vi "CANOpen_Main_Scale RPDO Data.vi"(8 "error in (no error)":errorcluster, 10 "Data":dbl[](array[numeric]), 11 "PDO Settings":T1={"Parameters"=[], "PDO Channel"=1, "Start Index"=0, "Length"=0} {"PDO Channel" items=["PDO 1", "PDO 2", "PDO 3", "PDO 4"]; "Parameters"."Bit Offset" max=8 step=1; "Parameters"."Byte Offset" max=8 step=1}) -> (0 "error out":errorcluster, 3 "CANopen data out":u8[](array[numeric]))   [LabVIEW 2013]
uses:
  Shared Code/CANOpen_PDO Settings.ctl
  Shared Code/CANOpen_PDO Parameter Settings.ctl
  Shared Code/CANOpen_PDO Data Type.ctl
  System Explorer/SubVIs/CANopen Byte Order.ctl
  <vilib>/CANopenLib/CANOPEN.llb/CANopen Convert To Data [U8].vi
  <vilib>/CANopenLib/CANOPEN.llb/CANopen Convert To Data [I8].vi
  <vilib>/CANopenLib/CANOPEN.llb/CANopen Convert To Data [I16].vi
  <vilib>/CANopenLib/CANOPEN.llb/CANopen Convert To Data [I32].vi
  <vilib>/CANopenLib/CANOPEN.llb/CANopen Convert To Data [SGL].vi
  <vilib>/CANopenLib/CANOPEN.llb/CANopen Convert To Data [DBL].vi
  <vilib>/CANopenLib/CANOPEN.llb/CANopen Convert To Data [U16].vi
  <vilib>/CANopenLib/CANOPEN.llb/CANopen Convert To Data [U32].vi
  CANOpen Addon Custom Device.lvlib
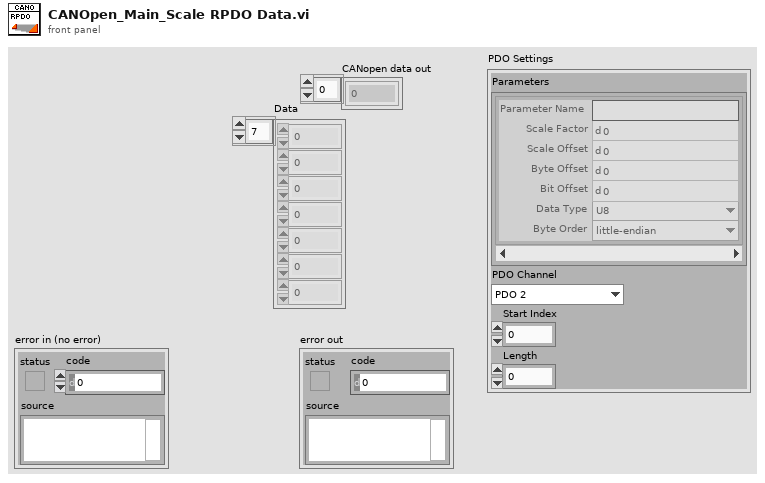
[diagram p1: front panel]
types:
  T1 = typedef "CANOpen Addon Custom Device.lvlib/CANOpen_PDO Settings.ctl" = cluster{"Parameters":T2[], "PDO Channel":u8, "Start Index":u32, "Length":u32}
  T2 = typedef "CANOpen Addon Custom Device.lvlib/CANOpen_PDO Parameter Settings.ctl" = cluster{"Parameter Name":string, "Scale Factor":dbl, "Scale Offset":dbl, "Byte Offset":u8, "Bit Offset":u8, "Data Type":T3, "Byte Order":T4}
  T3 = typedef "CANOpen Addon Custom Device.lvlib/CANOpen_PDO Data Type.ctl" = enum16{"U8", "U16", "U32", "I8", "I16", "I32", "Single", "Double", "Boolean"}
  T4 = typedef "CANOpen Addon Custom Device.lvlib/CANopen Byte Order.ctl" = enum16{"big-endian network order", "little-endian"}
  T5 = enum16{"big-endian, network order", "native, host order", "little-endian"}
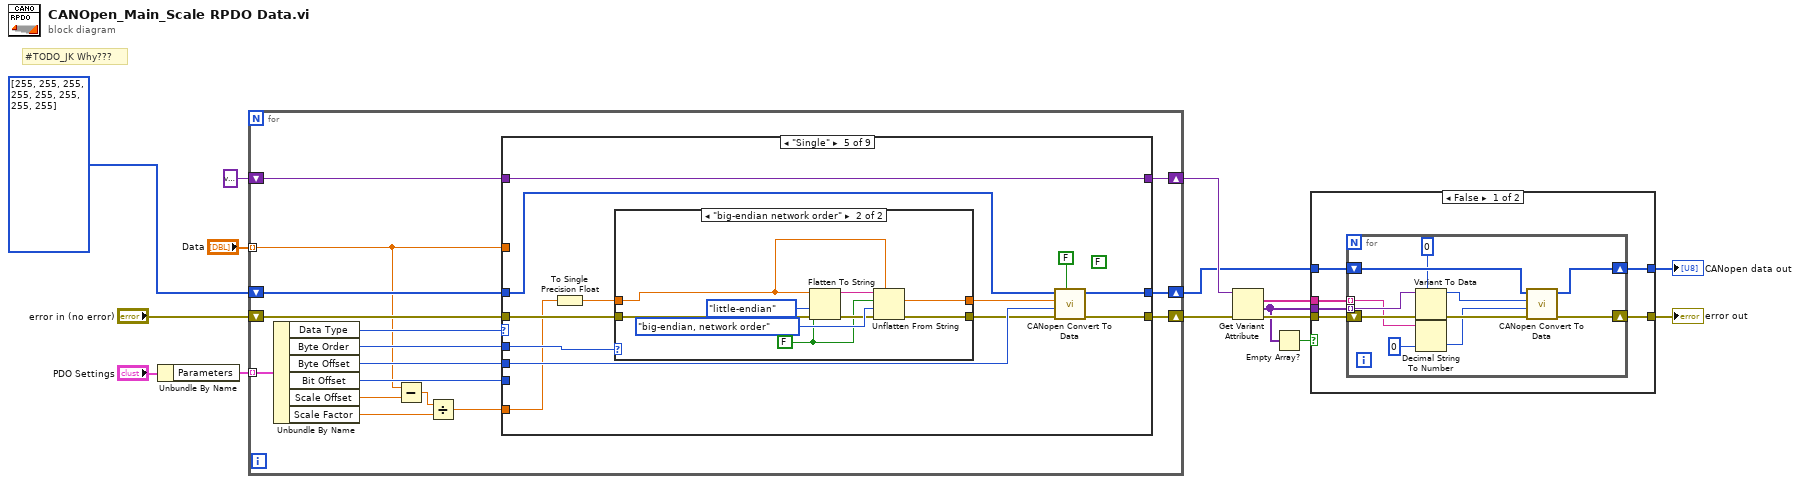
[diagram p0: block diagram]
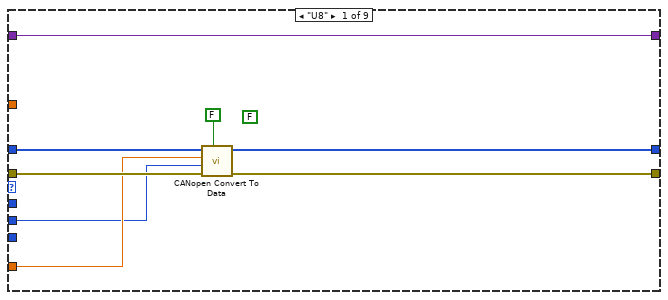
[diagram p3: hidden frame]
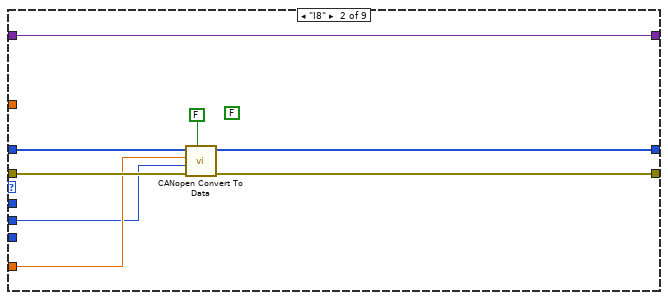
[diagram p4: hidden frame]
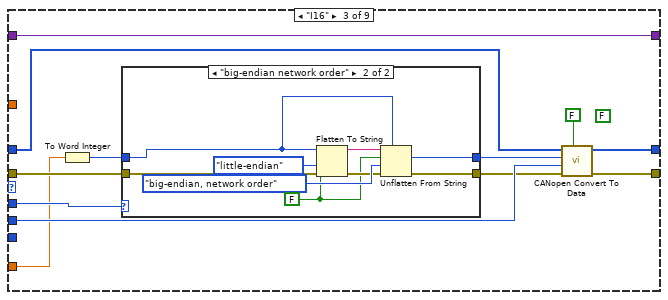
[diagram p5: hidden frame]
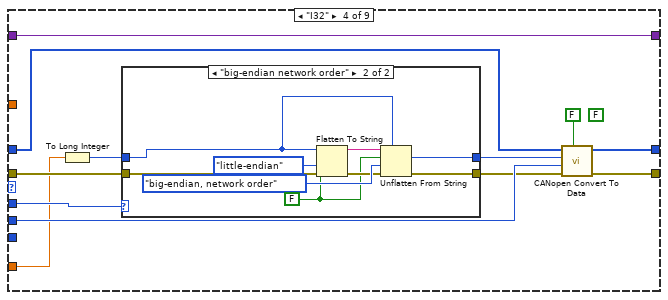
[diagram p7: hidden frame]
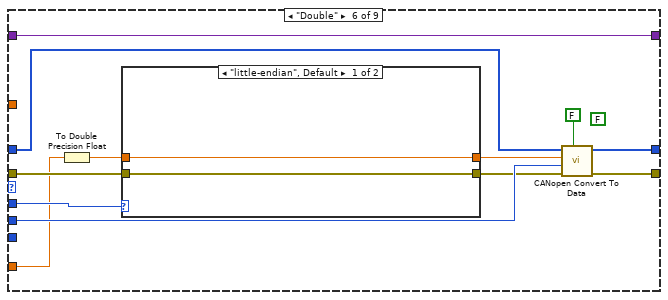
[diagram p10: hidden frame]
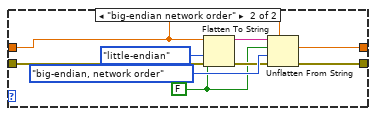
[diagram p11: hidden frame]
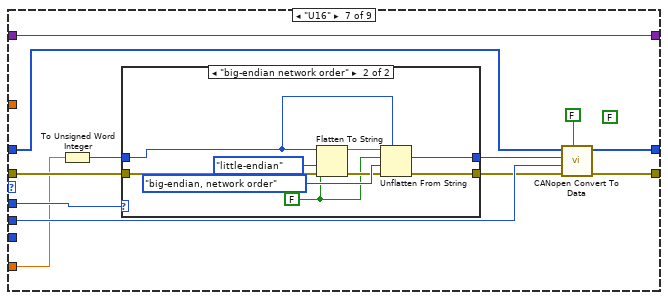
[diagram p12: hidden frame]
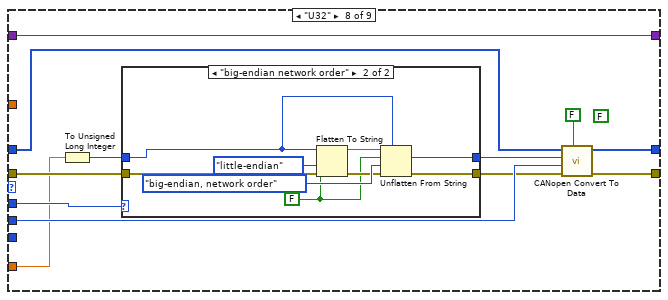
[diagram p14: hidden frame]
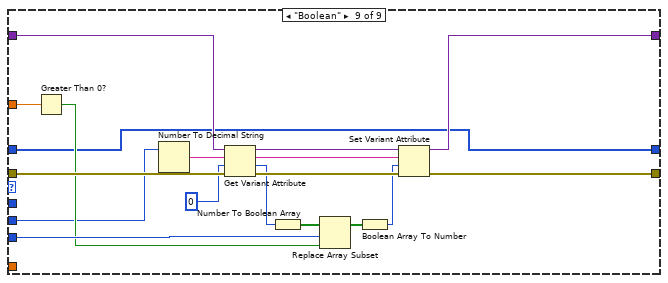
[diagram p16: hidden frame]
diagram:
  # "#TODO_JK Why???"
  n1 = Unbundle By Name("PDO Settings") -> ("Parameters"=w13:T2[])
  n2 = for {
    tunnel: w13 -> [w29] mode=indexing
    shift-right: [w23] -> w5
    shift-left: u8[] [255, 255, 255, 255, 255, 255, 255, 255] ("CANopen data out") -> [w22]
    shift-right: [w31] -> w10
    shift-left: "error in (no error)" -> [w30]
    shift-right: [w18] -> w9
    shift-left: variant ("variant") -> [w19]
    tunnel: "Data" -> [w16] mode=indexing
    n3 = Unbundle By Name(w29) -> ("Data Type"=w24:T3, "Byte Order"=w17:T4, "Byte Offset"=w25:u8, "Bit Offset"=w20:u8, "Scale Offset"=w28:dbl, "Scale Factor"=w21:dbl)
    n4 = Subtract(x=w16, y=w28) -> (x-y=w27:dbl)
    n5 = Divide(x=w27, y=w21) -> (x/y=w26:dbl)
    n6 = case shown="\"Single\"" w24 {
      tunnel: [w39 w47 w59 w82 w105 w128 w151 w174 w199] -> w31
      tunnel: [w37 w45 w57 w80 w103 w126 w149 w172 w189] -> w23
      tunnel: w30 -> [w36 w44 w54 w77 w100 w123 w146 w169 w201]
      tunnel: w26 -> [w35 w43 w49 w72 w95 w118 w141 w164 _]
      tunnel: w25 -> [w34 w42 w56 w79 w102 w125 w148 w171 w188]
      tunnel: w22 -> [w33 w41 w51 w74 w97 w120 w143 w166 w189]
      tunnel: w20 -> [_ _ _ _ _ _ _ _ w194]
      tunnel: w19 -> [w32 w40 w55 w78 w101 w124 w147 w170 w202]
      tunnel: [w32 w40 w55 w78 w101 w124 w147 w170 w190] -> w18
      tunnel: w17 -> [_ _ w52 w75 w98 w121 w144 w167 _]
      tunnel: w16 -> [_ _ _ _ _ _ _ _ w186]
      frame "U8" {
        (unwired) FALSE ("trim")
        n7 = call-poly <vilib>:"CANopen Convert To Data.vi"("trim"=FALSE, "error in (no error)"=w36, "offset (0)"=w34, "unsigned 8-bit integer"=w35, "CANopen data in"=w33) -> ("error out"=w39:errorcluster, "CANopen data out"=w37:u8[])  [unwired: 5 in]
      }
      frame "I8" {
        (unwired) FALSE ("trim")
        n8 = call-poly <vilib>:"CANopen Convert To Data.vi"("trim"=FALSE, "error in (no error)"=w44, "offset (0)"=w42, "signed 8-bit integer"=w43, "CANopen data in"=w41) -> ("error out"=w47:errorcluster, "CANopen data out"=w45:u8[])  [unwired: 5 in]
      }
      frame "I16" {
        (unwired) FALSE ("trim")
        n9 = To Word Integer(number=w49) -> (16bit integer=w50:i16)
        n10 = case shown="\"big-endian network order\"" w52 {
          tunnel: w50 -> [w60 w66]
          tunnel: [w60 w65] -> w48
          tunnel: w54 -> [w61 w64]
          tunnel: [w61 w63] -> w53
          frame "little-endian", Default {
          }
          frame "big-endian network order" {
            w62 = FALSE ("prepend array or string size? (T)")
            n11 = Flatten To String(anything=w66, prepend array or string size? (T)=w62, byte order (0:big-endian, network order)=T5."little-endian", error in (no error)=w64) -> (data string=w69:string, error out=w67:errorcluster)  [unwired: 1 out]
            n12 = Unflatten From String(type=w66, binary string=w69, data includes array or string size? (T)=w62, byte order (0:big-endian, network order)=T5."big-endian, network order", error in (no error)=w67) -> (value=w65:i16, error out=w63:errorcluster)  [unwired: 1 out]
          }
        }
        n13 = call-poly <vilib>:"CANopen Convert To Data.vi"("trim"=FALSE, "error in (no error)"=w53, "offset (0)"=w56, "signed 16-bit integer"=w48, "CANopen data in"=w51) -> ("error out"=w59:errorcluster, "CANopen data out"=w57:u8[])  [unwired: 5 in]
      }
      frame "I32" {
        (unwired) FALSE ("trim")
        n14 = To Long Integer(number=w72) -> (32bit integer=w73:i32)
        n15 = case shown="\"big-endian network order\"" w75 {
          tunnel: w73 -> [w83 w89]
          tunnel: [w83 w88] -> w71
          tunnel: w77 -> [w84 w87]
          tunnel: [w84 w86] -> w76
          frame "little-endian", Default {
          }
          frame "big-endian network order" {
            w85 = FALSE ("prepend array or string size? (T)")
            n16 = Flatten To String(anything=w89, prepend array or string size? (T)=w85, byte order (0:big-endian, network order)=T5."little-endian", error in (no error)=w87) -> (data string=w92:string, error out=w90:errorcluster)  [unwired: 1 out]
            n17 = Unflatten From String(type=w89, binary string=w92, data includes array or string size? (T)=w85, byte order (0:big-endian, network order)=T5."big-endian, network order", error in (no error)=w90) -> (value=w88:i32, error out=w86:errorcluster)  [unwired: 1 out]
          }
        }
        n18 = call-poly <vilib>:"CANopen Convert To Data.vi"("trim"=FALSE, "error in (no error)"=w76, "offset (0)"=w79, "signed 32-bit integer"=w71, "CANopen data in"=w74) -> ("error out"=w82:errorcluster, "CANopen data out"=w80:u8[])  [unwired: 5 in]
      }
      frame "Single" {
        (unwired) FALSE ("trim")
        n19 = To Single Precision Float(number=w95) -> (single precision float=w96:sgl)
        n20 = case shown="\"big-endian network order\"" w98 {
          tunnel: w96 -> [w106 w112]
          tunnel: [w106 w111] -> w94
          tunnel: w100 -> [w107 w110]
          tunnel: [w107 w109] -> w99
          frame "little-endian", Default {
          }
          frame "big-endian network order" {
            w108 = FALSE ("prepend array or string size? (T)")
            n21 = Flatten To String(anything=w112, prepend array or string size? (T)=w108, byte order (0:big-endian, network order)=T5."little-endian", error in (no error)=w110) -> (data string=w115:string, error out=w113:errorcluster)  [unwired: 1 out]
            n22 = Unflatten From String(type=w112, binary string=w115, data includes array or string size? (T)=w108, byte order (0:big-endian, network order)=T5."big-endian, network order", error in (no error)=w113) -> (value=w111:sgl, error out=w109:errorcluster)  [unwired: 1 out]
          }
        }
        n23 = call-poly <vilib>:"CANopen Convert To Data.vi"("trim"=FALSE, "error in (no error)"=w99, "offset (0)"=w102, "4-byte single"=w94, "CANopen data in"=w97) -> ("error out"=w105:errorcluster, "CANopen data out"=w103:u8[])  [unwired: 5 in]
      }
      frame "Double" {
        (unwired) FALSE ("trim")
        n24 = To Double Precision Float(number=w118) -> (double precision float=w119:dbl)
        n25 = case shown="\"little-endian\", Default" w121 {
          tunnel: w119 -> [w129 w135]
          tunnel: [w129 w134] -> w117
          tunnel: w123 -> [w130 w133]
          tunnel: [w130 w132] -> w122
          frame "little-endian", Default {
          }
          frame "big-endian network order" {
            w131 = FALSE ("prepend array or string size? (T)")
            n26 = Flatten To String(anything=w135, prepend array or string size? (T)=w131, byte order (0:big-endian, network order)=T5."little-endian", error in (no error)=w133) -> (data string=w138:string, error out=w136:errorcluster)  [unwired: 1 out]
            n27 = Unflatten From String(type=w135, binary string=w138, data includes array or string size? (T)=w131, byte order (0:big-endian, network order)=T5."big-endian, network order", error in (no error)=w136) -> (value=w134:dbl, error out=w132:errorcluster)  [unwired: 1 out]
          }
        }
        n28 = call-poly <vilib>:"CANopen Convert To Data.vi"("trim"=FALSE, "error in (no error)"=w122, "offset (0)"=w125, "8-byte double"=w117, "CANopen data in"=w120) -> ("error out"=w128:errorcluster, "CANopen data out"=w126:u8[])  [unwired: 5 in]
      }
      frame "U16" {
        (unwired) FALSE ("trim")
        n29 = To Unsigned Word Integer(number=w141) -> (unsigned 16bit integer=w142:u16)
        n30 = case shown="\"big-endian network order\"" w144 {
          tunnel: w142 -> [w152 w158]
          tunnel: [w152 w157] -> w140
          tunnel: w146 -> [w153 w156]
          tunnel: [w153 w155] -> w145
          frame "little-endian", Default {
          }
          frame "big-endian network order" {
            w154 = FALSE ("prepend array or string size? (T)")
            n31 = Flatten To String(anything=w158, prepend array or string size? (T)=w154, byte order (0:big-endian, network order)=T5."little-endian", error in (no error)=w156) -> (data string=w161:string, error out=w159:errorcluster)  [unwired: 1 out]
            n32 = Unflatten From String(type=w158, binary string=w161, data includes array or string size? (T)=w154, byte order (0:big-endian, network order)=T5."big-endian, network order", error in (no error)=w159) -> (value=w157:u16, error out=w155:errorcluster)  [unwired: 1 out]
          }
        }
        n33 = call-poly <vilib>:"CANopen Convert To Data.vi"("trim"=FALSE, "error in (no error)"=w145, "offset (0)"=w148, "unsigned 16-bit integer"=w140, "CANopen data in"=w143) -> ("error out"=w151:errorcluster, "CANopen data out"=w149:u8[])  [unwired: 5 in]
      }
      frame "U32" {
        (unwired) FALSE ("trim")
        n34 = To Unsigned Long Integer(number=w164) -> (unsigned 32bit integer=w165:u32)
        n35 = case shown="\"big-endian network order\"" w167 {
          tunnel: w165 -> [w175 w181]
          tunnel: [w175 w180] -> w163
          tunnel: w169 -> [w176 w179]
          tunnel: [w176 w178] -> w168
          frame "little-endian", Default {
          }
          frame "big-endian network order" {
            w177 = FALSE ("prepend array or string size? (T)")
            n36 = Flatten To String(anything=w181, prepend array or string size? (T)=w177, byte order (0:big-endian, network order)=T5."little-endian", error in (no error)=w179) -> (data string=w184:string, error out=w182:errorcluster)  [unwired: 1 out]
            n37 = Unflatten From String(type=w181, binary string=w184, data includes array or string size? (T)=w177, byte order (0:big-endian, network order)=T5."big-endian, network order", error in (no error)=w182) -> (value=w180:u32, error out=w178:errorcluster)  [unwired: 1 out]
          }
        }
        n38 = call-poly <vilib>:"CANopen Convert To Data.vi"("trim"=FALSE, "error in (no error)"=w168, "offset (0)"=w171, "unsigned 32-bit integer"=w163, "CANopen data in"=w166) -> ("error out"=w174:errorcluster, "CANopen data out"=w172:u8[])  [unwired: 5 in]
      }
      frame "Boolean" {
        n39 = Greater Than 0?(x=w186) -> (x > 0?=w193:bool)
        n40 = Number To Decimal String(number=w188) -> (decimal integer string=w187:string)  [unwired: 1 in]
        n41 = Get Variant Attribute(Variant=w202, name=w187, default value (empty Variant)=u8 0, error in=w201) -> (duplicate Variant=w198:variant, value=w196:u8, error out=w200:errorcluster)  [unwired: 1 out]
        n42 = Number To Boolean Array(number=w196) -> (Boolean array=w195:bool[])
        n43 = Replace Array Subset(array=w195, new element=w193, index=w194) -> (w192:bool[])
        n44 = Boolean Array To Number(Boolean array=w192) -> (number=w191:u32)
        n45 = Set Variant Attribute(Variant=w198, name=w187, value=w191, error in=w200) -> (Variant out=w190:variant, error out=w199:errorcluster)  [unwired: 1 out]
      }
    }
  }
  n46 = Get Variant Attribute(Variant=w9, error in=w10) -> (names=w3:string[], values=w2:variant[], error out=w8:errorcluster)  [unwired: 2 in, 1 out]
  n47 = Empty Array?(array=w2) -> (empty?=w6:bool)
  n48 = case shown="False" w6 {
    tunnel: w8 -> [w208 w221]
    tunnel: [w207 w221] -> w7
    tunnel: w5 -> [w206 w220]
    tunnel: [w205 w220] -> w4
    tunnel: w3 -> [w204 _]
    tunnel: w2 -> [w203 _]
    frame False {
      n49 = for {
        shift-right: [w217] -> w205
        shift-left: w206 -> [w218]
        shift-right: [w219] -> w207
        shift-left: w208 -> [w216]
        tunnel: w204 -> [w211] mode=indexing
        tunnel: w203 -> [w214] mode=indexing
        n50 = Variant To Data(error in=w216, type=u8 0, Variant=w214) -> (data=w212:u8, error out=w215:errorcluster)
        n51 = Decimal String To Number(string=w211, default (0L)=u8 0 ("Byte Offset")) -> (number=w209:u8)  [unwired: 1 in, 1 out]
        n52 = call-poly <vilib>:"CANopen Convert To Data.vi"("error in (no error)"=w215, "offset (0)"=w209, "unsigned 8-bit integer"=w212, "CANopen data in"=w218) -> ("error out"=w219:errorcluster, "CANopen data out"=w217:u8[])  [unwired: 6 in]
      }
    }
    frame True {
    }
  }
  "CANopen data out" <- w4
  "error out" <- w7
